vi "test_libssh2_version.vi"() -> ()   [LabVIEW 2013, in "libssh2_tests.lvlib"]
uses:
  libssh2/libssh2_init_default.vi
  libssh2_tests.lvlib
  libssh2/libssh2.lvlib
  <vilib>/addons/_JKI Toolkits/Caraya/classes/Test/Test.lvclass
  Assert Extensions/Assert Extensions.lvclass
panel:
  out "error out":errorcluster
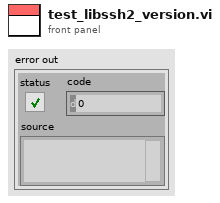
[diagram p1: front panel]
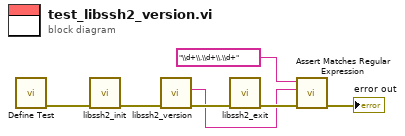
[diagram p0: block diagram]
diagram:
  n1 = call <vilib>:"Define Test.vi"() -> ("error out"=w3:errorcluster)  [unwired: 10 in, 1 out]
  n2 = call-poly "libssh2_init.vi"("error in (no error)"=w3) -> ("error out"=w7:errorcluster)  [unwired: 10 in]
  n3 = call "libssh2_version.vi"("error in (no error)"=w7) -> ("error out"=w5:errorcluster, "version"=w1:string)  [unwired: 9 in]
  n4 = call "libssh2_exit.vi"("error in (no error)"=w5) -> ("error out"=w6:errorcluster)  [unwired: 10 in]
  n5 = call "Assert Matches Regular Expression.vi"("error in (no error)"=w6, "Actual Value"=w1, "Regular Expression"="\\d+\\.\\d+\\.\\d+") -> ("error out"=→"error out":errorcluster)  [unwired: 8 in]
